vi "queryValue.vi"(8 "error in (no error)":errorcluster, 10 "queries":T1, 11 "DomeController in":refnum<class "DomeController.lvclass">) -> (0 "error out":errorcluster, 2 "Variant":variant, 3 "DomeController out":refnum<class "DomeController.lvclass">)   [LabVIEW 2016, in "DomeController.lvclass"]
uses:
  DomeController.lvclass
  domeCommunicator/ComTypedefs/queries.ctl
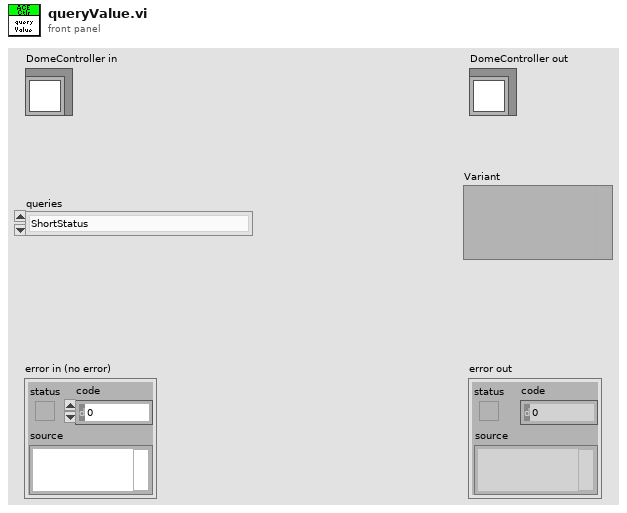
[diagram p1: front panel]
types:
  T1 = typedef "queries.ctl" = enum16{"ShortStatus", "FullEngineeringStatus", "RecallLastSavedConfiguration"}
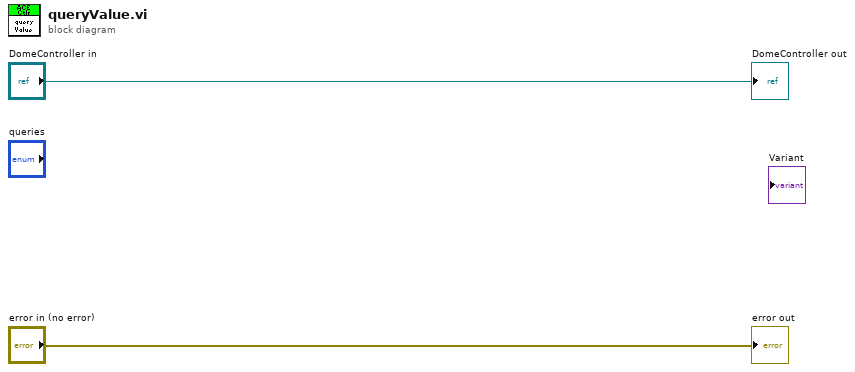
[diagram p0: block diagram]
diagram:
  "error out" <- "error in (no error)"
  "DomeController out" <- "DomeController in"
